vi "AcquireData.vi"() -> (3 "Data Graph":dynamicdata(graph))   [LabVIEW 2014]
uses:
  <vilib>/Platform/storage/lvStorage.llb/xStorage/xStorageSupp/ErrorOut.vi
  <vilib>/Platform/storage/lvStorage.llb/xStorage/Open Data Storage/Open Data Storage.xnode
  <vilib>/Platform/storage/lvStorage.llb/xStorage/Read Data/Read Data.xnode
  <vilib>/Platform/storage/lvStorage.llb/xStorage/Close Data Storage/Close Data Storage.xnode
  <vilib>/Platform/storage/lvStorage.llb/_openStorageWithRootAutoDetect.vi
  <vilib>/Platform/storage/lvStorage.llb/_openFunction.ctl
  <vilib>/Platform/storage/lvStorage.llb/_defaultFilePath.vi
  <vilib>/Platform/storage/lvStorage.llb/_queryPropPoly.vi
  <vilib>/Platform/storage/lvStorage.llb/_queryPropString.vi
  <vilib>/Platform/storage/lvStorage.llb/_queryGenericObjects.vi
  <vilib>/Platform/storage/lvStorage.llb/_loadAllDdt.vi
  <vilib>/Platform/storage/Storage.llb/Get Object Info.vi
  <vilib>/Platform/storage/Storage.llb/__closeStorageFromObject.vi
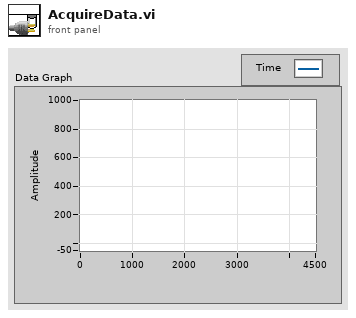
[diagram p1: front panel]
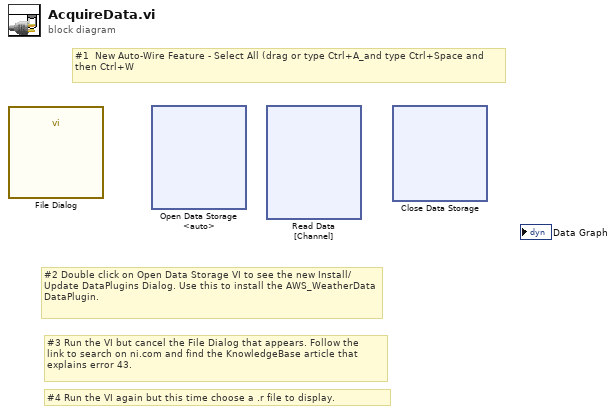
[diagram p0: block diagram]
diagram:
  # "#4 Run the VI again but this time choose a .r file to display."
  # "#3 Run the VI but cancel the File Dialog that appears. Follow the\nlink to search on ni.com and find the KnowledgeBase article that\nexplains error 43."
  # "#2 Double click on Open Data Storage VI to see the new Install/Update DataPlugins Dialog. Use this to install the AWS_WeatherData DataPlugin."
  # "#1  New Auto-Wire Feature - Select All (drag or type Ctrl+A_and type Ctrl+Space and then Ctrl+W"
  n1 = call "File Dialog"() -> ()  [unwired: 12 in, 4 out]
  n2 = xnode "Open Data Storage\n<auto>"() -> ()  [unwired: 5 in, 3 out]
  n3 = xnode "Read Data\n[Channel]"() -> ()  [unwired: 4 in, 4 out]
  n4 = xnode "Close Data Storage\n"() -> ()  [unwired: 2 in, 2 out]
